vi "Persist Config.vi"(8 "error in (no error)":errorcluster, 10 "Root":refnum<class "Config Element.lvclass">, 11 "Config-YAML in":refnum<class "Config-YAML.lvclass">) -> (0 "error out":errorcluster, 3 "Config-YAML out":refnum<class "Config-YAML.lvclass">)   [LabVIEW 2020, in "CDM-Config.lvlib" / "Config-YAML.lvclass"]
uses:
  Config-YAML.lvclass
  Config Element/Config Element.lvclass
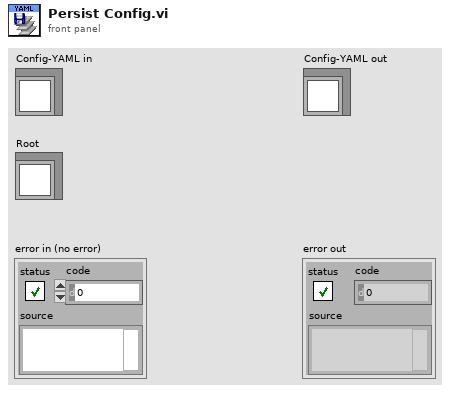
[diagram p1: front panel]
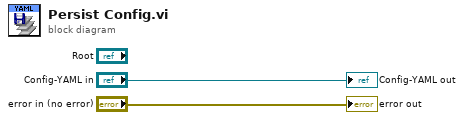
[diagram p0: block diagram]
diagram:
  "error out" <- "error in (no error)"
  "Config-YAML out" <- "Config-YAML in"
